vi "RichToFlatpumploop_SetControlRequest.vi"(5 "OutputClusterType":T1, 11 "InputCluster":T3) -> (3 "OutputCluster":T1)   [LabVIEW 2024, in "pumploop_client.lvlib"]
uses:
  pumploop_client.lvlib
  pumploop_SetControlRequest.ctl
  pumploop_Controls.ctl
  pumploop_SetControlRequest_Flat.ctl
  pumploop_Controls_Flat.ctl
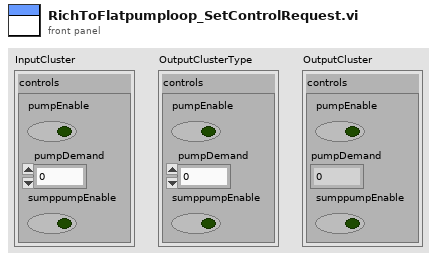
[diagram p1: front panel]
types:
  T1 = typedef "pumploop_client.lvlib/pumploop_SetControlRequest_Flat.ctl" = cluster{"controls":T2}
  T2 = typedef "pumploop_client.lvlib/pumploop_Controls_Flat.ctl" = cluster{"pumpEnable":bool, "pumpDemand":sgl, "sumppumpEnable":bool}
  T3 = typedef "pumploop_client.lvlib/pumploop_SetControlRequest.ctl" = cluster{"controls":T4}
  T4 = typedef "pumploop_client.lvlib/pumploop_Controls.ctl" = cluster{"pumpEnable":bool, "pumpDemand":sgl, "sumppumpEnable":bool}
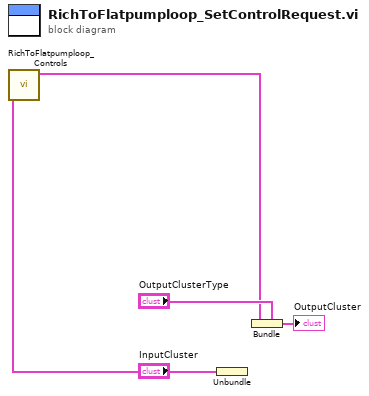
[diagram p0: block diagram]
diagram:
  n1 = Unbundle "Unbundle"("InputCluster") -> ("controls"=w2:T4)
  n2 = call "RichToFlatpumploop_Controls.vi"("InputCluster"=w2) -> ("OutputCluster"=w1:T2)  [unwired: 10 in]
  n3 = Bundle "Bundle"(cluster="OutputClusterType", "controls"=w1) -> (→"OutputCluster":T1)
